vi "samples write (host with fpga).vi"(5 "channel number":u32=1, 6 "trigger to write samples":bool, 7 "samples per packet":u32=1000, 9 "number of packets to detect":u32, 10 "file for writing samples":refnum<file>, 11 "fpga cluster":T1 {"Daughterboard Clock Rate" format="%#.3pHz"; "FPGA Data Clock Rate" format="%#.3pHz"; "Data Clock Rate" format="%#.3pHz"; "Characterization Data"."Frequencies [Hz]" format="%#_6p"; "EEPROM Characterization Header"."Pointer to Device Data Header" format="%x"; "EEPROM Characterization Header"."Checksum" format="%x"; "Device Data Header"."Pointer to Characterization Data" format="%x"; "Device Data Header"."Checksum" format="%x"; "EEPROM Header"."Pointer to User Header" format="%x"; "EEPROM Header"."Pointer to Factory Header" format="%x"; "EEPROM Header"."Product Code" format="%x"; "EEPROM Header"."Checksum" format="%x"}) -> (1 "samples num":u32, 2 "samples is written":bool, 3 "samples":string)   [LabVIEW 2020]
uses:
  <instrlib>/niUsrpRio/Config/v1/Host/Public/niUsrpRio Session.ctl
  <instrlib>/_niInstr/Register Bus/v0/Host/Public/Register Bus Session.ctl
  <instrlib>/_niInstr/Register Bus/v0/Host/Private/Session Data.ctl
  <instrlib>/niUsrpRio/Config/v1/Host/Private/DB Queue Reference.ctl
  <instrlib>/niUsrpRio/Config/v1/Host/Private/Daughterboard Data.ctl
  <instrlib>/niUsrpRio/Config/v1/Host/Private/ATR state data.ctl
  <instrlib>/niUsrpRio/Config/v1/Host/Private/Antenna Configuration.ctl
  <instrlib>/niUsrpRio/Config/v1/Host/Private/CPLD Power Mode.ctl
  <instrlib>/niUsrpRio/Config/v1/Host/Public/EEPROM Header.ctl
  <instrlib>/niUsrpRio/Config/v1/Host/Public/EEPROM Device Data Header.ctl
  <instrlib>/niUsrpRio/Config/v1/Host/Public/EEPROM Characterization Header.ctl
  <instrlib>/niUsrpRio/Config/v1/Host/Public/Characterization Data.ctl
  <instrlib>/niUsrpRio/Config/v1/Host/Public/IQ Imbalance.ctl
  Host/SubVIs/Streaming Xvcr FPGA Ref.ctl
  <vilib>/rvi/interface/common/niFpgaWaitOnOcc.vi
  <vilib>/Utility/error.llb/Error Cluster From Error Code.vi
  <vilib>/rvi/errors/niLvFpgaAdjustHostInterfaceError.vi
  <vilib>/rvi/interface/nirviMethod/nirviMethod.xnode
  <vilib>/rvi/errors/niLvFpgaMergeErrorWithErrorCode.vi
  <vilib>/FPGAPlugInAG/Dynamic/niLvFpga_ReadFifo_Dynamic.vi
  <vilib>/FPGAPlugInAG/Dynamic/niLvFpga_ConfigureFifo_Dynamic.vi
  <instrlib>/_niInstr/Register Bus/v0/Host/niInstr Register Bus v0 Host.lvlib
  <instrlib>/niUsrpRio/Config/v1/Host/niUsrpRio Config v1 Host.lvlib
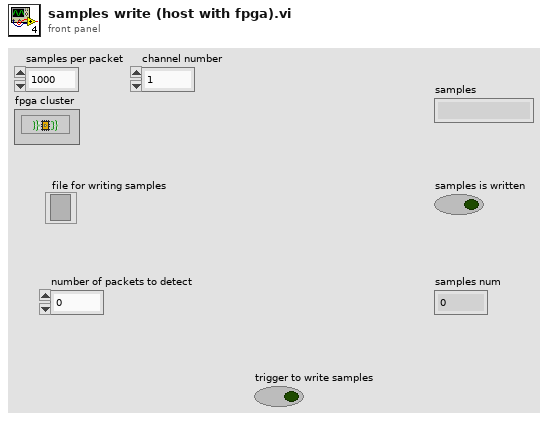
[diagram p1: front panel]
types:
  T1 = typedef "niUsrpRio Config v1 Host.lvlib/niUsrpRio Session.ctl" = cluster{"FPGA Interface":refnum<k20>, "RIO Interface Number":u32, "Data Clock Rate":u32, "FPGA Data Clock Rate":u32, "Global Settings Register Bus":T2, "Radio 0 Settings Register Bus":T2, "Radio 1 Settings Register Bus":T2, "Radio Settings Bus Semaphore":T3, "DB Queues":T4[], "Characterization Data Valid?":bool, "EEPROM Header":T5, "Device Data Header":T6, "EEPROM Characterization Header":T7, "Characterization Data":T8[], "FPGA Current Version":u32, "FPGA Oldest Compatible Version":u32, "Fixed Logic Current Version":u32, "Fixed Logic Oldest Compatible Version":u32, "FPGA Radio Settings Bus Current Version":u32, "FPGA Radio Settings Bus Oldest Compatible Version":u32, "FPGA Board Config Current Version":u32, "FPGA Board Config Oldest Compatible Version":u32, "Daughterboard Clock Rate":u32, "daughterboard configuration session handles":u64[]}
  T2 = typedef "niInstr Register Bus v0 Host.lvlib/Register Bus Session.ctl" = refnum<queue>
  T3 = typedef "Semaphore RefNum" = refnum<k1>
  T4 = typedef "niUsrpRio Config v1 Host.lvlib/DB Queue Reference.ctl" = refnum<queue>
  T5 = typedef "niUsrpRio Config v1 Host.lvlib/EEPROM Header.ctl" = cluster{"Checksum":u32, "Product Code":u16, "Hardware Current Version":u16, "Hardware Oldest Compatible Version":u16, "EEPROM Map Current Version":u16, "EEPROM Map Oldest Compatible Version":u16, "User Password":string, "Pointer to Factory Header":u32, "Pointer to User Header":u32, "Recommended Interval":u16, "Number of Reserved Bytes":i32, "Number of Daughterboards":u8, "Daughterboard IDs":u16[], "Daughterboard Serial Numbers":string[]}
  T6 = typedef "niUsrpRio Config v1 Host.lvlib/EEPROM Device Data Header.ctl" = cluster{"Checksum":u32, "Number of Channels":u8, "Number of Gain Settings":u16[], "Pointer to Characterization Data":u32[], "Number of Reserved Bytes":i32, "Number of Frequencies":u16[]}
  T7 = typedef "niUsrpRio Config v1 Host.lvlib/EEPROM Characterization Header.ctl" = cluster{"Checksum":u32, "Date":timestamp, "Temperature":sgl, "Misc. Info":string, "Pointer to Device Data Header":u32, "Number of Reserved Bytes":i32}
  T8 = typedef "niUsrpRio Config v1 Host.lvlib/Characterization Data.ctl" = cluster{"Gains[dB]":dbl[], "Frequencies [Hz]":dbl[], "IQ Imbalance Table":T9[], "Measured Gains[dB]":dbl[][]}
  T9 = typedef "niUsrpRio Config v1 Host.lvlib/IQ Imbalance.ctl" = cluster{"Gain Imbalance [linear]":dbl, "Phase Imbalance [radians]":dbl, "Offset":cdb}
  T10 = typedef "Streaming Xvcr FPGA Ref.ctl" = refnum<k20>
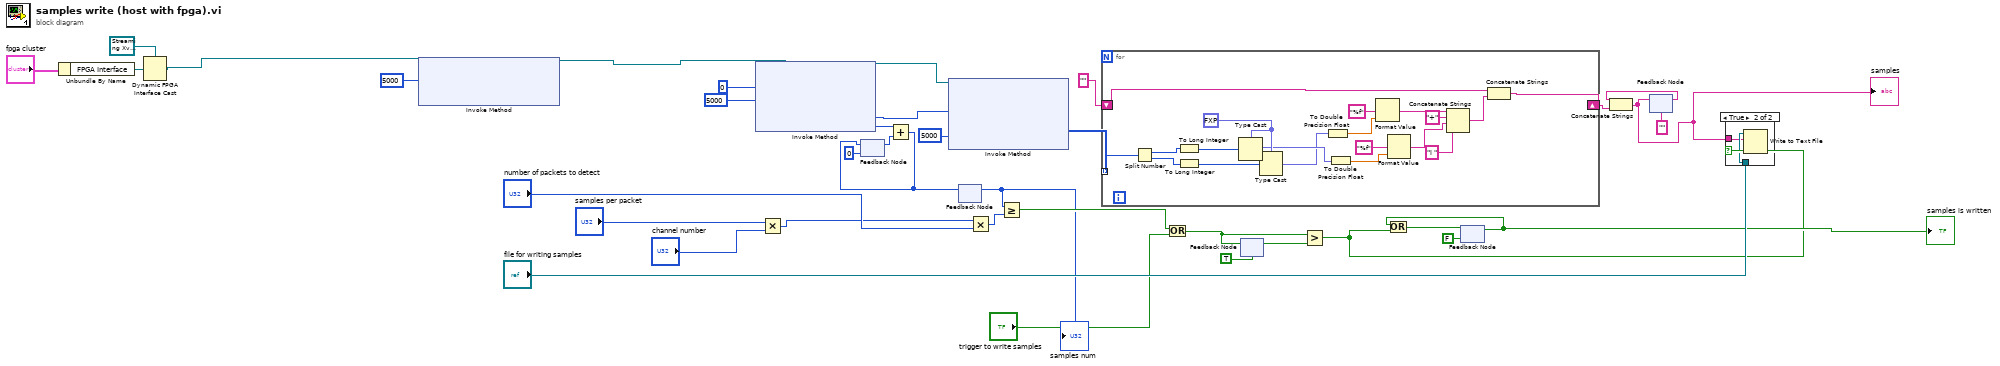
[diagram p0: block diagram]
diagram:
  n1 = Unbundle By Name("fpga cluster") -> ("FPGA Interface"=w4:refnum<k20>)
  n2 = Dynamic FPGA Interface Cast(Session In=T10 refnum ("Type"), Type=w4) -> (Session Out=w2:T10)
  n3 = xnode "Invoke Method"("FPGA VI Reference In"=w2, "Requested Depth"=u32 5000) -> ("FPGA VI Reference Out"=w5:T10)  [unwired: 1 in, 2 out]
  n4 = xnode "Invoke Method"("FPGA VI Reference In"=w5, "Number of Elements"=u32 0, "Timeout (ms)"=5000) -> ("FPGA VI Reference Out"=w18:T10, "Elements Remaining"=w23:u32)  [unwired: 1 in, 2 out]
  n5 = Multiply(x="samples per packet", y="channel number") -> (x*y=w6:u32)
  n6 = feedback #1(u32 0) -> (w22:u32)
  n7 = Add(x=w23, y=w22) -> (x+y=w25:u32)
  n8 = feedback-in #1(w25) -> ()
  n9 = xnode "Invoke Method"("FPGA VI Reference In"=w18, "Number of Elements"=w23, "Timeout (ms)"=5000) -> ("Data"=w16:u64[])  [unwired: 1 in, 3 out]
  n10 = feedback #2() -> (w29:u32)  [unwired: 1 in]
  "samples num" <- w29
  n11 = feedback-in #2(w25) -> ()
  n12 = Multiply(x=w6, y="number of packets to detect") -> (x*y=w28:u32)
  n13 = Greater Or Equal?(x=w29, y=w28) -> (x >= y?=w31:bool)
  n14 = for {
    tunnel: w16 -> [w42] mode=indexing
    shift-right: [w37] -> w17
    shift-left: "" -> [w39]
    w52 = fxp<+/-,32,11> 0.0 ("Number of Elements")
    n15 = Split Number(x=w42) -> (hi(x)=w55:u32, lo(x)=w54:u32)
    n16 = To Long Integer(number=w55) -> (32bit integer=w53:i32)
    n17 = To Long Integer(number=w54) -> (32bit integer=w41:i32)
    n18 = Type Cast(type=w52, x=w53) -> (*(type *) &x=w50:fxp<+/-,32,11>)
    n19 = Type Cast(type=w52, x=w41) -> (*(type *) &x=w40:fxp<+/-,32,11>)
    n20 = To Double Precision Float(number=w40) -> (double precision float=w49:dbl)
    n21 = To Double Precision Float(number=w50) -> (double precision float=w47:dbl)
    n22 = Format Value(format string="%f", value (0)=w49) -> (output string=w46:string)  [unwired: 1 in]
    n23 = Format Value(format string="%f", value (0)=w47) -> (output string=w44:string)  [unwired: 1 in]
    n24 = Concatenate Strings(w46, "+" ("string"), w44, "i " ("string")) -> (w38:string)
    n25 = Concatenate Strings(w39, w38) -> (w37:string)
  }
  n26 = Or(x=w31, y="trigger to write samples") -> (x .or. y?=w27:bool)
  n27 = feedback #3(TRUE ("trigger to write csi and samples")) -> (w20:bool)
  n28 = feedback-in #3(w27) -> ()
  n29 = Greater?(x=w27, y=w20) -> (0:w34:bool)
  n30 = feedback #4(FALSE) -> (w35:bool)
  "samples is written" <- w35
  n31 = Or(x=w35, y=w34) -> (x .or. y?=w33:bool)
  n32 = feedback-in #4(w33) -> ()
  n33 = feedback #5("" ("output string")) -> (w14:string)
  n34 = Concatenate Strings(w14, w17) -> (w15:string)
  "samples" <- w15
  n35 = feedback-in #5(w15) -> ()
  n36 = case shown="True" w34 {
    tunnel: "file for writing samples" -> [_ w57]
    tunnel: w15 -> [_ w56]
    frame False {
    }
    frame True {
      n37 = Write to Text File(file (use dialog)=w57, text=w56) -> ()  [unwired: 2 in, 3 out]
    }
  }
